vi "GrabBackground.vi"() -> ()   [LabVIEW 2011]
uses:
  <vilib>/vision/Image Controls.llb/IMAQ Image.ctl
  Main/Camera/CIGrabParams.ctl
  qtrk/QTrkLVBinding/QTrkInstance.ctl
  qtrk/QTrkLVBinding/ResultManagerInstance.ctl
  Main/Camera/CIGrabControlMsg.ctl
  Main/Camera/CIGrabControlMsgEnum.ctl
  Main/GlobalVariables.vi
  <vilib>/vision/NI_Vision_Development_Module.lvlib
panel:
  out "Image-Background":T1(plugin-control)
  in  "Export path":path=path "D:/jcnossen1/qtrk/bin/mc1362_background.bin"
  in  "F_a":sgl=0.002
  in  "Save":bool
  out "Tmp Img":T1
  out "Background":T1(plugin-control)
  in  "Grab loop":bool
  out "Frame #":i32
  out "Image":T1(plugin-control)
  in  "Grab Framerate (Hz)":i32=20
  in  "Grab background":bool
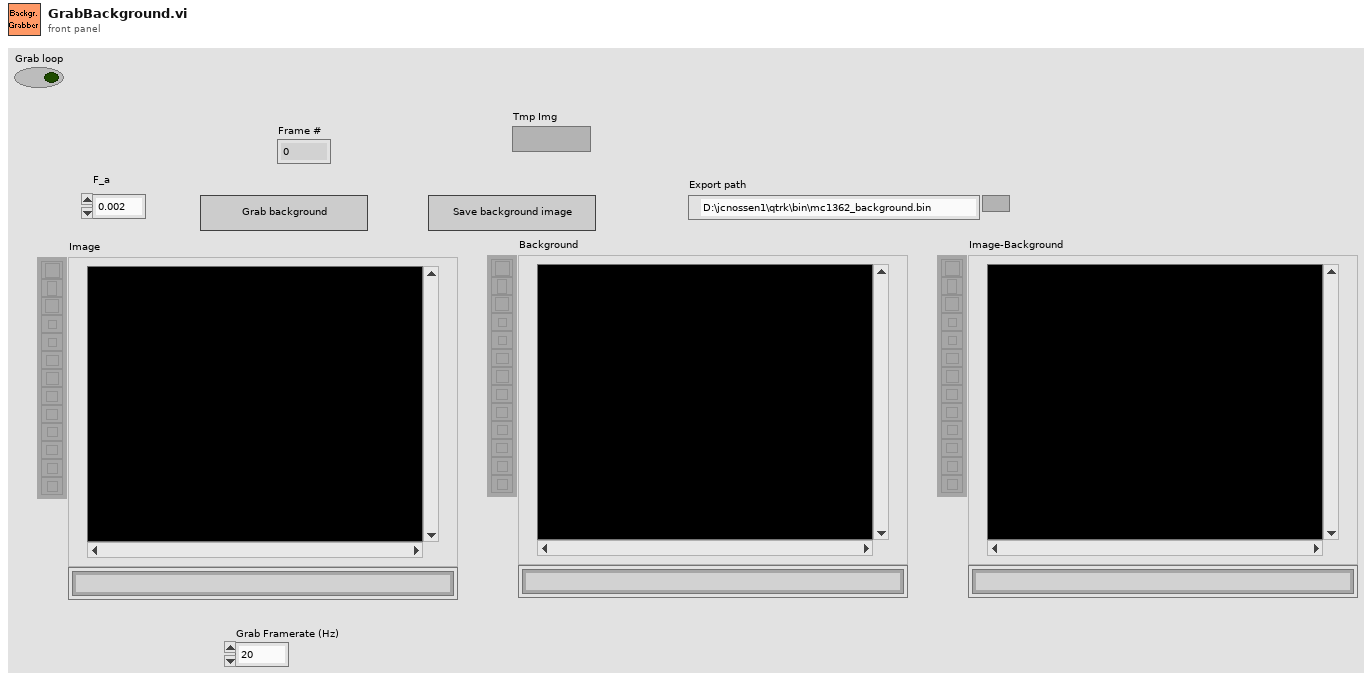
[diagram p1: front panel]
types:
  T1 = typedef "IMAQ Image.ctl" = refnum<image>
  T2 = typedef "Image Type" = u32
  T3 = enum16{"big-endian, network order", "native, host order", "little-endian"}
  T4 = typedef "CIGrabParams.ctl" = cluster{"QTrk Instance":T5, "ResultManager":T6, "Send to queue?":bool, "Force full-frame capture":bool}
  T5 = typedef "QTrkInstance.ctl" = cluster{"QTrk Pointer":u64}
  T6 = typedef "ResultManagerInstance.ctl" = cluster{"InstancePtr":u64}
  T7 = typedef "CIGrabControlMsg.ctl" = cluster{"Msg":T8}
  T8 = typedef "CIGrabControlMsgEnum.ctl" = enum16{"Stop", "EnableTracking", "DisableTracking"}
  T9 = typedef "CIGrabType.ctl" = refnum<vi>
  T10 = typedef "CmdData_NewFrame.ctl" = cluster{"Buffer Image":T1, "Frame #":i32, "Hardware ROI Index":i32, "Timestamp":dbl, "Type":T11}
  T11 = typedef "CmdEnum_CameraFrameType.ctl" = enum16{"Full", "HardwareROI", "EndGrabMarker"}
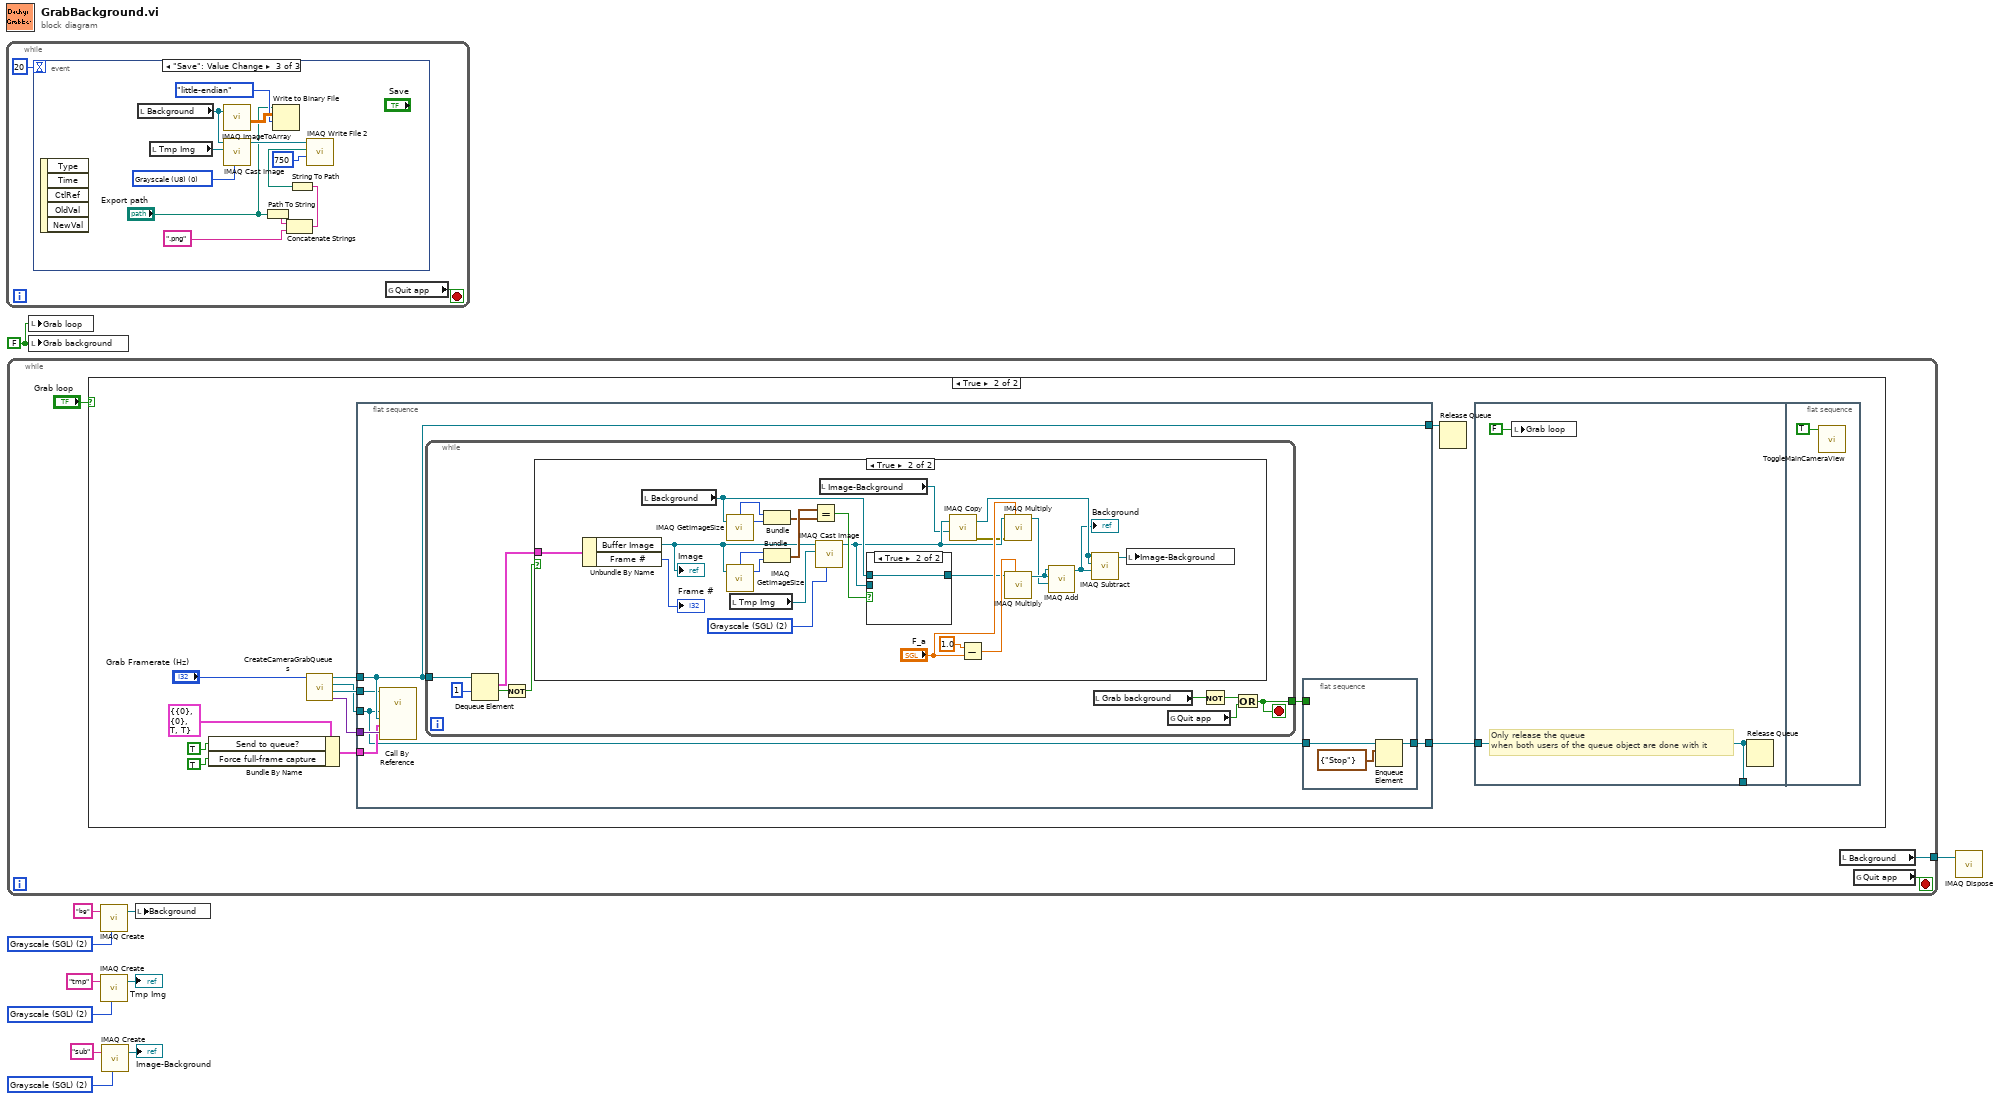
[diagram p0: block diagram]
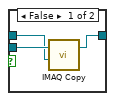
[diagram p4: hidden frame]
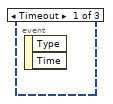
[diagram p5: hidden frame]
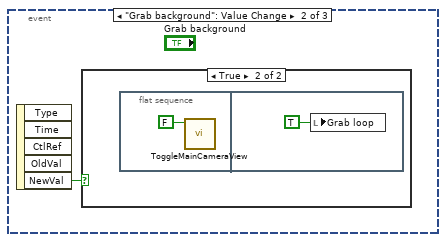
[diagram p6: hidden frame]
diagram:
  w3 = T2 2 items=["Grayscale (U8)", "Grayscale (I16)", "Grayscale (SGL)", "Complex (CSG)", "RGB (U32)", "HSL (U32)", "RGB (U64)", "Grayscale (U16)"] ("Image Type")
  w4 = T2 2 items=["Grayscale (U8)", "Grayscale (I16)", "Grayscale (SGL)", "Complex (CSG)", "RGB (U32)", "HSL (U32)", "RGB (U64)", "Grayscale (U16)"] ("Image Type")
  w5 = T2 2 items=["Grayscale (U8)", "Grayscale (I16)", "Grayscale (SGL)", "Complex (CSG)", "RGB (U32)", "HSL (U32)", "RGB (U64)", "Grayscale (U16)"] ("Image Type")
  w11 = FALSE ("Grab background")
  n1 = while {
    stop <- w13 stop-if-true
    n2 = event shown="[2] \"Save\": Value Change" {
      selector: _ -> [_ _ _]
      dyn-events: _ -> [_ _ _]
      timeout: 20 -> [_ _ _]
      event Timeout {
        n3 = event-data() -> ()  [unwired: 1 in, 2 out]
      }
      event "Grab background": Value Change {
        n4 = event-data() -> ("NewVal"=w14:bool)  [unwired: 1 in, 4 out]
        n5 = case shown="True" w14 {
          frame False {
          }
          frame True {
            n6 = flat-sequence {
              frame #0 {
                n7 = call "ToggleMainCameraView.vi"("Enable? (T)"=FALSE) -> ()  [unwired: 11 in]
              }
              frame #1 {
                n8 = local write "Grab loop"(TRUE ("Grab loop")) -> ()
              }
            }
          }
        }
      }
      event "Save": Value Change {
        w26 = T2 0 items=["Grayscale (U8)", "Grayscale (I16)", "Grayscale (SGL)", "Complex (CSG)", "RGB (U32)", "HSL (U32)", "RGB (U64)", "Grayscale (U16)"] ("Image Type")
        n9 = event-data() -> ()  [unwired: 1 in, 5 out]
        n10 = local read "Background"() -> (w24:T1)
        n11 = local read "Tmp Img"() -> (w27:T1)
        n12 = call "IMAQ ImageToArray"("Image"=w24) -> ("Image Pixels (Float)"=w23:sgl[][])  [unwired: 3 in, 4 out]
        n13 = call "IMAQ Cast Image"("Image Type"=w26, "Image Dst"=w27, "Image Src"=w24) -> ("Image Dst Out"=w25:T1)  [unwired: 7 in, 1 out]
        n14 = Path To String(path="Export path") -> (string=w20:string)
        n15 = Write to Binary File(file (use dialog)="Export path", data=w23, 9:T3."little-endian" ("byte order (0:big-endian, network order)")) -> ()  [unwired: 3 in, 3 out]
        n16 = Concatenate Strings(w20, ".png" ("name or relative path")) -> (w18:string)
        n17 = String To Path(string=w18) -> (path=w17:path)
        n18 = call-poly "IMAQ Write File 2"("Image Quality"=u32 750, "File Path"=w17, "Image"=w25) -> ()  [unwired: 7 in, 2 out]
      }
    }
    n19 = global read "GlobalVariables.vi" "Quit app"() -> (w13:bool)
  }
  n20 = while {
    tunnel: [w29] -> w8
    stop <- w31 stop-if-true
    n21 = case shown="True" "Grab loop" {
      frame False {
      }
      frame True {
        n22 = Bundle By Name(cluster=T4 {"QTrk Instance"={"QTrk Pointer"=0}, "ResultManager"={"InstancePtr"=0}, "Send to queue?"=TRUE, "Force full-frame capture"=TRUE} ("TrackingParameters"), "Send to queue?"=TRUE, "Force full-frame capture"=TRUE) -> (w34:T4)
        n23 = call "CreateCameraGrabQueues.vi"("Framerate (Hz)"="Grab Framerate (Hz)") -> ("Camera state (out)"=w40:variant, "VI refs.Grab"=w41:T9, "GrabControlQueue"=w33:refnum<queue>, "CameraOutQueue"=w39:refnum<queue>)  [unwired: 7 in]
        n24 = flat-sequence {
          tunnel: [w52] -> w38
          tunnel: [w51] -> w32
          tunnel: w33 -> [w46]
          tunnel: w34 -> [w48]
          tunnel: w39 -> [w52]
          tunnel: w40 -> [w49]
          tunnel: w41 -> [w50]
          frame #0 {
            n25 = call-by-ref "?"(reference=w50, "Camera data"=w49, "TrackingParameters"=w48, "Output Queue"=w52, "GrabControlQueue"=w46) -> ()  [unwired: 8 in, 3 out]
            n26 = while {
              tunnel: w52 -> [w60]
              tunnel: [w56] -> w47
              stop <- w56 stop-if-true
              n27 = Dequeue Element(queue=w60, timeout in ms (-1)=1) -> (element=w63:T10, timed out?=w62:bool)  [unwired: 1 in, 2 out]
              n28 = Not(x=w62) -> (.not. x?=w61:bool)
              n29 = case shown="True" w61 {
                tunnel: w63 -> [_ w89]
                frame False {
                }
                frame True {
                  w81 = T2 2 items=["Grayscale (U8)", "Grayscale (I16)", "Grayscale (SGL)", "Complex (CSG)", "RGB (U32)", "HSL (U32)", "RGB (U64)", "Grayscale (U16)"] ("Image Type")
                  n30 = Unbundle By Name(w89) -> ("Buffer Image"=w80:T1, "Frame #"=→"Frame #":i32)
                  "Image" <- w80
                  n31 = local read "Background"() -> (w77:T1)
                  n32 = call "IMAQ GetImageSize"("Image"=w77) -> ("Y Resolution"=w84:i32, "X Resolution"=w85:i32)  [unwired: 3 in, 1 out]
                  n33 = call "IMAQ GetImageSize"("Image"=w80) -> ("Y Resolution"=w86:i32, "X Resolution"=w87:i32)  [unwired: 3 in, 1 out]
                  n34 = local read "Tmp Img"() -> (w79:T1)
                  n35 = Bundle("X Resolution"=w85, "Y Resolution"=w84) -> (w82:cluster{"X Resolution":i32, "Y Resolution":i32})  [unwired: 1 in]
                  n36 = Bundle("X Resolution"=w87, "Y Resolution"=w86) -> (w83:cluster{"X Resolution":i32, "Y Resolution":i32})  [unwired: 1 in]
                  n37 = Equal?(x=w83, y=w82) -> (x = y?=w78:bool)
                  n38 = call "IMAQ Cast Image"("Image Type"=w81, "Image Dst"=w79, "Image Src"=w80) -> ("Image Dst Out"=w70:T1)  [unwired: 7 in, 1 out]
                  n39 = local read "Image-Background"() -> (w69:T1)
                  n40 = case shown="True" w78 {
                    tunnel: w70 -> [w92 _]
                    tunnel: w77 -> [w91 w93]
                    tunnel: [w90 w93] -> w73
                    frame False {
                      n41 = call "IMAQ Copy"("Image Dst"=w91, "Image Src"=w92) -> ("Image Dst Out"=w90:T1)  [unwired: 4 in, 1 out]
                    }
                    frame True {
                    }
                  }
                  n42 = call "IMAQ Copy"("Image Dst"=w69, "Image Src"=w70) -> ("error out"=w68:errorcluster, "Image Dst Out"=w67:T1)  [unwired: 4 in]
                  n43 = Subtract(x=1.0, y="F_a") -> (x-y=w74:dbl)
                  n44 = call "IMAQ Multiply"("Image Src A"=w70, "Constant"="F_a", "error in (no error)"=w68) -> ("Image Dst Out"=w71:T1)  [unwired: 4 in, 1 out]
                  n45 = call "IMAQ Multiply"("Image Src A"=w73, "Constant"=w74) -> ("Image Dst Out"=w72:T1)  [unwired: 5 in, 1 out]
                  n46 = call "IMAQ Add"("Image Src A"=w72, "Image Dst"=w72, "Image Src B"=w71) -> ("Image Dst Out"=w66:T1)  [unwired: 4 in, 1 out]
                  "Background" <- w66
                  n47 = call "IMAQ Subtract"("Image Src A"=w67, "Image Dst"=w67, "Image Src B"=w66) -> ("Image Dst Out"=w65:T1)  [unwired: 4 in, 1 out]
                  n48 = local write "Image-Background"(w65) -> ()
                }
              }
              n49 = local read "Grab background"() -> (w59:bool)
              n50 = global read "GlobalVariables.vi" "Quit app"() -> (w58:bool)
              n51 = Not(x=w59) -> (.not. x?=w57:bool)
              n52 = Or(x=w57, y=w58) -> (x .or. y?=w56:bool)
            }
            n53 = flat-sequence {
              tunnel: w47 -> [_]
              tunnel: w46 -> [w54]
              tunnel: [w53] -> w51
              frame #0 {
                n54 = Enqueue Element(queue=w54, element=T7 {"Msg"=enum."Stop"}) -> (queue out=w53:refnum<queue>)  [unwired: 2 in, 2 out]
              }
            }
          }
        }
        n55 = Release Queue(queue=w38) -> ()  [unwired: 2 in, 3 out]
        n56 = flat-sequence {
          tunnel: [w43] -> _
          tunnel: w32 -> [w43]
          frame #0 {
            # "Only release the queue\nwhen both users of the queue object are done with it"
            n57 = local write "Grab loop"(FALSE ("Grab loop")) -> ()
            n58 = Release Queue(queue=w43) -> ()  [unwired: 2 in, 3 out]
          }
          frame #1 {
            n59 = call "ToggleMainCameraView.vi"("Enable? (T)"=TRUE) -> ()  [unwired: 11 in]
          }
        }
      }
    }
    n60 = local read "Background"() -> (w29:T1)
    n61 = global read "GlobalVariables.vi" "Quit app"() -> (w31:bool)
  }
  n62 = local write "Grab loop"(w11) -> ()
  n63 = local write "Grab background"(w11) -> ()
  n64 = call "IMAQ Create"("Image Name"="bg", "Image Type"=w4) -> ("New Image"=w10:T1)  [unwired: 3 in, 1 out]
  n65 = call "IMAQ Create"("Image Name"="tmp", "Image Type"=w5) -> ("New Image"=→"Tmp Img":T1)  [unwired: 3 in, 1 out]
  n66 = call "IMAQ Create"("Image Name"="sub", "Image Type"=w3) -> ("New Image"=→"Image-Background":T1)  [unwired: 3 in, 1 out]
  n67 = local write "Background"(w10) -> ()
  n68 = call "IMAQ Dispose"("Image"=w8) -> ()  [unwired: 5 in, 1 out]
